vi "GetCustomData.vi"(8 "error in":errorcluster, 11 "FailureReference in":refnum<class "FailureReference.lvclass">) -> (0 "error out":errorcluster, 2 "CustomData":refnum<class "CustomData.lvclass">, 3 "FailureReference out":refnum<class "FailureReference.lvclass">)   [LabVIEW 2021, in "ProligentXMLGenerator.lvlib" / "FailureReference.lvclass"]
doc: "Get CustomData\n\nThe values defined under this element will not be interpreted by the DIT. It can be used to store data that will be used by another system."
uses:
  FailureReference.lvclass
  FailureReference.lvclass/FailureReference.ctl
  Model/CustomData/CustomData.lvclass
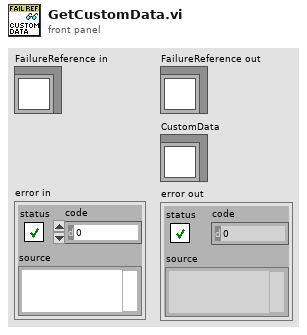
[diagram p1: front panel]
types:
  T1 = typedef "ProligentXMLGenerator.lvlib/FailureReference.lvclass/Data.ctl" = cluster{"Name":string, "CustomData":refnum<class "CustomData.lvclass">, "Id":refnum<class "Guid.lvclass">}
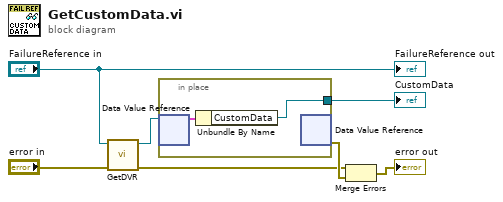
[diagram p0: block diagram]
diagram:
  n1 = call "GetDVR.vi"("error in"="error in", "FailureReference in"="FailureReference in") -> ("error out"=w1:errorcluster, "DVRReference"=w6:refnum<data-value>)  [unwired: 8 in]
  n2 = in-place "In Place Element Structure" {
    in-place-border: [w8] -> w2
    n3 = in-place-dvr #1(w6) -> (w9:T1)  [unwired: 1 out]
    n4 = Unbundle By Name(w9) -> ("CustomData"=w8:refnum<class "CustomData.lvclass">)
    n5 = in-place-dvr #1() -> (w7:errorcluster)  [unwired: 1 in, 1 out]
  }
  "CustomData" <- w2
  n6 = Merge Errors(w1, w7) -> (→"error out":errorcluster)
  "FailureReference out" <- "FailureReference in"
